vi "Update Overall Result.vi"(9 "Data Row":i32, 10 "Position":u32, 11 "Application in":refnum<class "Application.lvclass">) -> (3 "Pass":bool)   [LabVIEW 2017, in "Application.lvlib" / "Application.lvclass"]
uses:
  Application.lvclass
  <vilib>/TSS/ACRObat Test Framework/Core Launcher/Core Manager Methods -- Enum.ctl
  <vilib>/TSS/ACRObat Test Framework/Classes/Data/Data Repo/Class/Data Repo.lvclass
  <vilib>/TSS/ACRObat Test Framework/Core Launcher/Core Launcher.lvlib
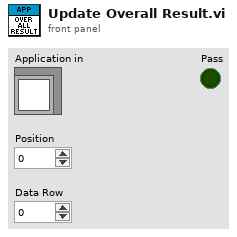
[diagram p1: front panel]
types:
  T1 = typedef "Core Launcher.lvlib/Core Manager Methods -- Enum.ctl" = enum16{"Spawn Objects", "Get Objects", "Destroy Objects"}
  T2 = typedef "Application.lvlib/App Properties.lvclass/Test Result -- Cluster.ctl" = cluster{"Position":i32, "Pass":bool, "Fail Codes":string}
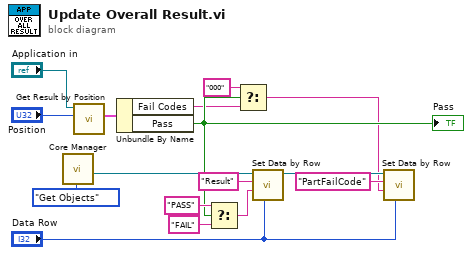
[diagram p0: block diagram]
diagram:
  n1 = call <vilib>:"Core Manager.vi"("Method"=Core_Manager_Methods_--_Enum."Get Objects") -> ("Data Repo"=w8:refnum<class "Data Repo.lvclass">)  [unwired: 6 in, 4 out]
  n2 = call "Get Result by Position.vi"("Position"="Position", "Application in"="Application in") -> ("Test Results"=w16:T2)  [unwired: 8 in, 1 out]
  n3 = Unbundle By Name(w16) -> ("Fail Codes"=w3:string, "Pass"=w4:bool)
  "Pass" <- w4
  n4 = Select(t="PASS", s=w4, f="FAIL") -> (s? t:f=w13:string)
  n5 = Select(t="000", s=w4, f=w3) -> (s? t:f=w1:string)
  n6 = call <vilib>:"Set Data by Row.vi"("Row"="Data Row", "Value"=w13, "Header"="Result", "Acrobat Template in"=w8) -> ("Acrobat Template out"=w6:refnum<class "Data Repo.lvclass">)  [unwired: 6 in, 1 out]
  n7 = call <vilib>:"Set Data by Row.vi"("Row"="Data Row", "Value"=w1, "Header"="PartFailCode", "Acrobat Template in"=w6) -> ()  [unwired: 6 in, 2 out]
